vi "batch_length.vi"(11 "preregistraion_data":T1) -> (3 "batch_length":i32)   [LabVIEW 2018]
uses:
  controls/preregistration_data.ctl
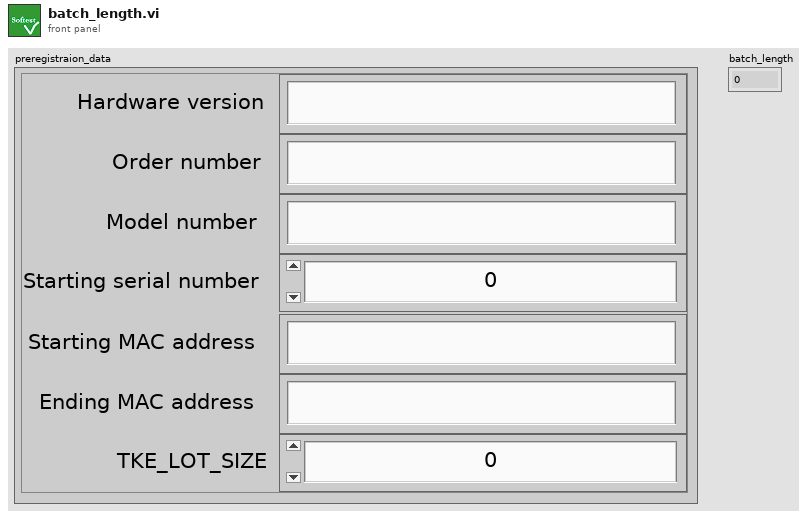
[diagram p1: front panel]
types:
  T1 = typedef "preregistration_data.ctl" = cluster{"Hardware version":string, "Order number":string, "Model number":string, "Starting serial number":i32, "Starting MAC address":string, "Ending MAC address":string, "TKE_LOT_SIZE":i32}
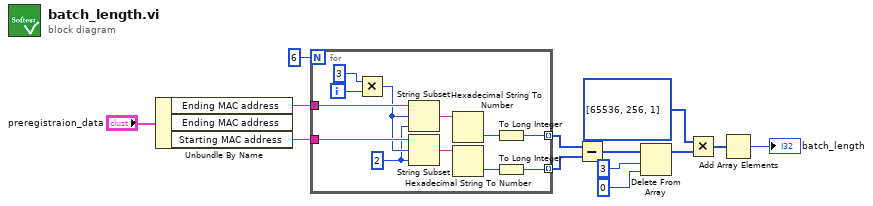
[diagram p0: block diagram]
diagram:
  n1 = Unbundle By Name("preregistraion_data") -> ("Ending MAC address"=w4:string, "Starting MAC address"=w3:string)  [unwired: 1 out]
  n2 = for {
    N: 6 -> [_]
    tunnel: w3 -> [w25]
    tunnel: w4 -> [w22]
    tunnel: [w15] -> w5 mode=indexing
    tunnel: [w14] -> w6 mode=indexing
    i -> [w24]
    w20 = 2 ("length (rest)")
    n3 = Multiply(x=3, y=w24) -> (x*y=w21:i32)
    n4 = String Subset(string=w22, offset (0)=w21, length (rest)=w20) -> (substring=w19:string)
    n5 = String Subset(string=w25, offset (0)=w21, length (rest)=w20) -> (substring=w18:string)
    n6 = Hexadecimal String To Number(string=w19) -> (number=w17:u32)  [unwired: 2 in, 1 out]
    n7 = Hexadecimal String To Number(string=w18) -> (number=w16:u32)  [unwired: 2 in, 1 out]
    n8 = To Long Integer(number=w17) -> (32bit integer=w15:i32)
    n9 = To Long Integer(number=w16) -> (32bit integer=w14:i32)
  }
  n10 = Subtract(x=w5, y=w6) -> (x-y=w7:i32[])
  n11 = Delete From Array(array=w7, length=3, index=0) -> (array with subset deleted=w11:i32[])  [unwired: 1 out]
  n12 = Multiply(x=i32[] [65536, 256, 1], y=w11) -> (x*y=w12:i32[])
  n13 = Add Array Elements(numeric array=w12) -> (sum=→"batch_length":i32)
